vi "SensorScaling.vi"(0 "Temperature Voltage (V)":dbl, 5 "Current Voltage (V)":dbl, 7 "Torque Voltage (V)":dbl, 9 "Vibration Voltage (V)":dbl, 11 "RPM Voltage (V)":dbl) -> (4 "Temperature (°C)":dbl, 6 "Current (A)":dbl, 8 "Torque (Nm)":dbl, 10 "Vibration (mm/s)":dbl, 15 "Actual RPM":dbl)   [LabVIEW 2026]
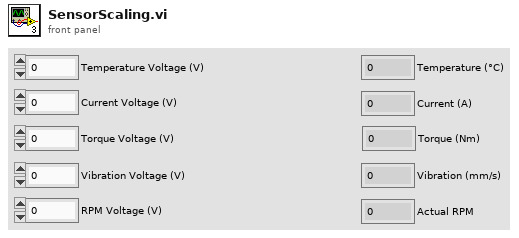
[diagram p1: front panel]
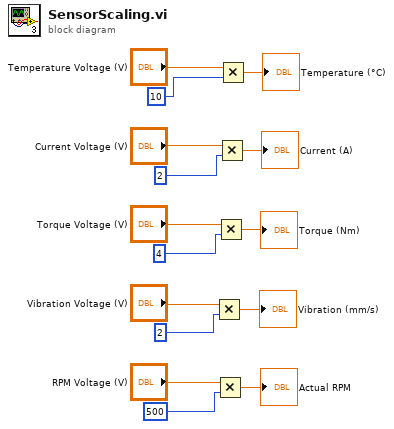
[diagram p0: block diagram]
diagram:
  n1 = Multiply(x="Vibration Voltage (V)", y=2) -> (x*y=→"Vibration (mm/s)":dbl)
  n2 = Multiply(x="RPM Voltage (V)", y=500) -> (x*y=→"Actual RPM":dbl)
  n3 = Multiply(x="Torque Voltage (V)", y=4) -> (x*y=→"Torque (Nm)":dbl)
  n4 = Multiply(x="Current Voltage (V)", y=2) -> (x*y=→"Current (A)":dbl)
  n5 = Multiply(x="Temperature Voltage (V)", y=10) -> (x*y=→"Temperature (°C)":dbl)
